vi "build_polymorphic_queues.vi"(2 "object/interaction_cluster_paths (in)":path[](array[path]), 5 "error in (no error)":errorcluster, 7 "base_federate_dir (in)":path, 8 "status_ref (in)":refnum<vi>) -> (19 "error out":errorcluster)   [LabVIEW 2016]
uses:
  controls/build_polymorphic_queues_actions.ctl
  <vilib>/picture/picture.llb/imagedata.ctl
  <vilib>/Utility/miscctls.llb/LVPositionTypeDef.ctl
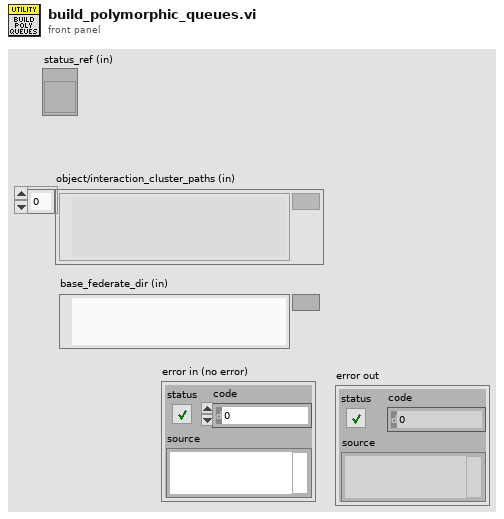
[diagram p1: front panel]
types:
  T1 = typedef "build_polymorphic_queues_actions.ctl" = enum16{"--------- unused ---------", "create_poly_instances", "create_poly_queues", "init"}
  T2 = typedef "imagedata.ctl" = cluster{"image type":i32, "image depth":i32, "image":u8[], "mask":u8[], "colors":u32[], "Rectangle":cluster{"left":i16, "top":i16, "right":i16, "bottom":i16}}
  T3 = enum32{"invalid app kind", "Development System", "Run Time System", "Student Edition", "Embedded LabVIEW", "Evaluation", "Custom"}
  T4 = typedef "LVPositionTypeDef.ctl" = cluster{"Left":i32, "Top":i32}
  T5 = enum32{"invalid VI type", "Standard VI", "Control VI", "Global VI", "Polymorphic VI", "Configuration VI", "SubSystem", "Facade VI", "Method VI", "Statechart Diagram VI"}
  T6 = cluster{"VIPath":path, "Menu Name":string, "Selector Name":string}
  T7 = cluster{"VIPath":path, "Menu Name":string, "Selector Name":string}[][]
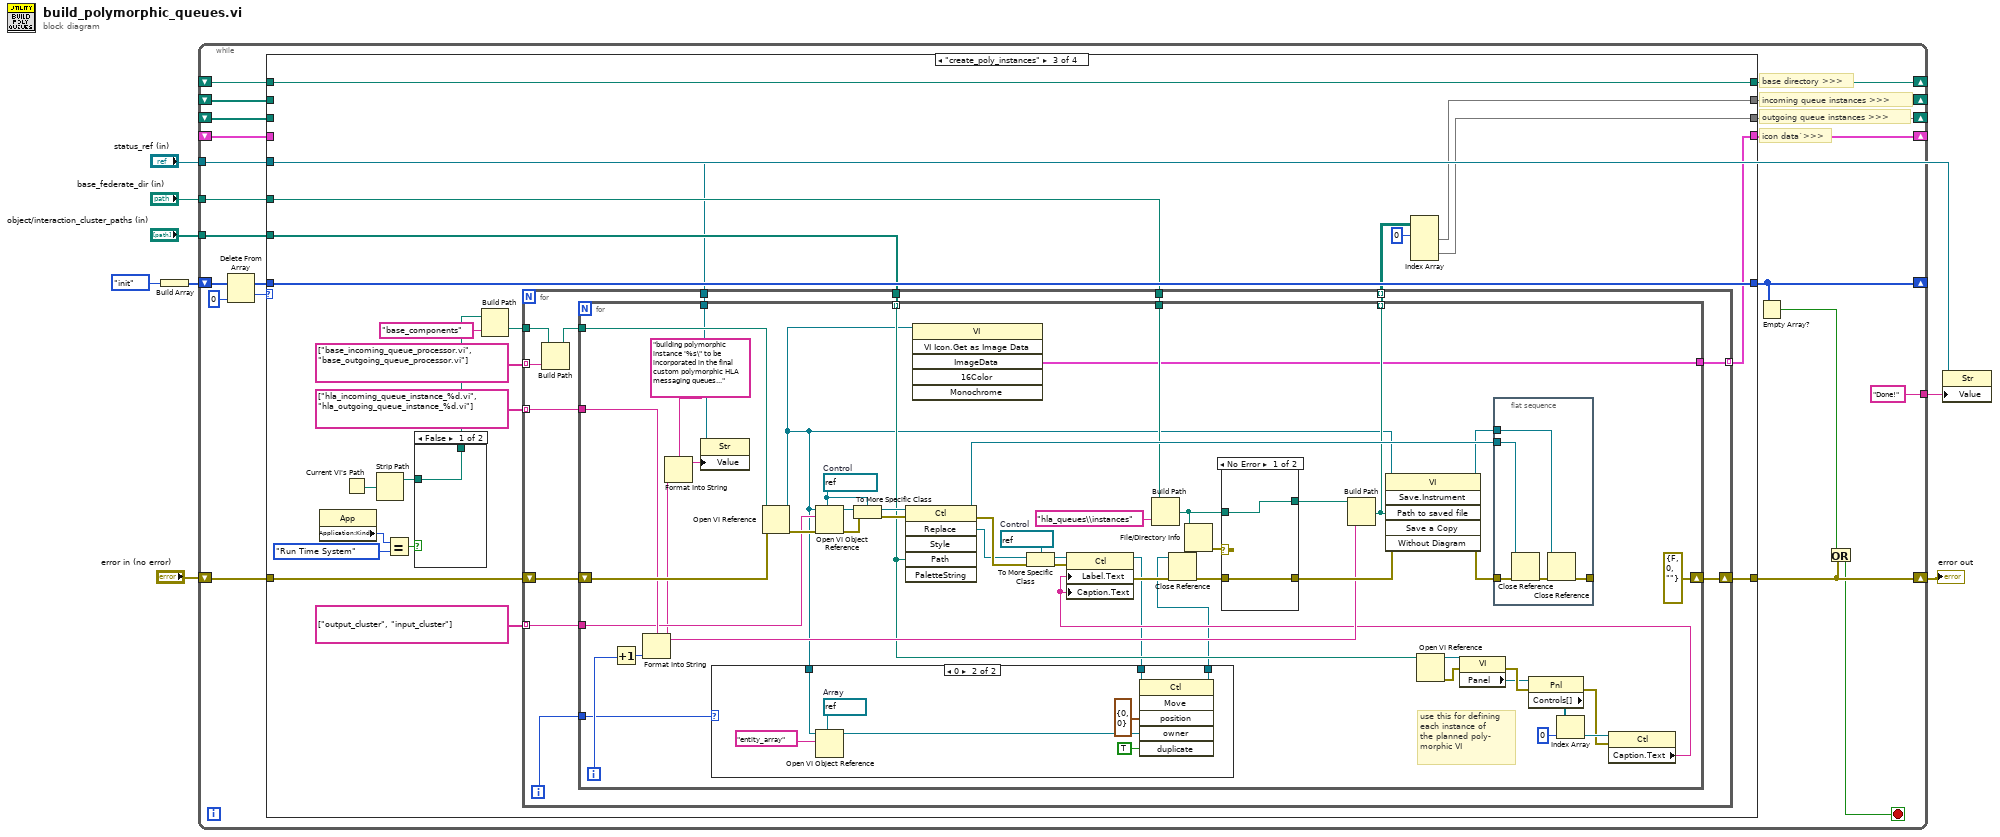
[diagram p0: block diagram]
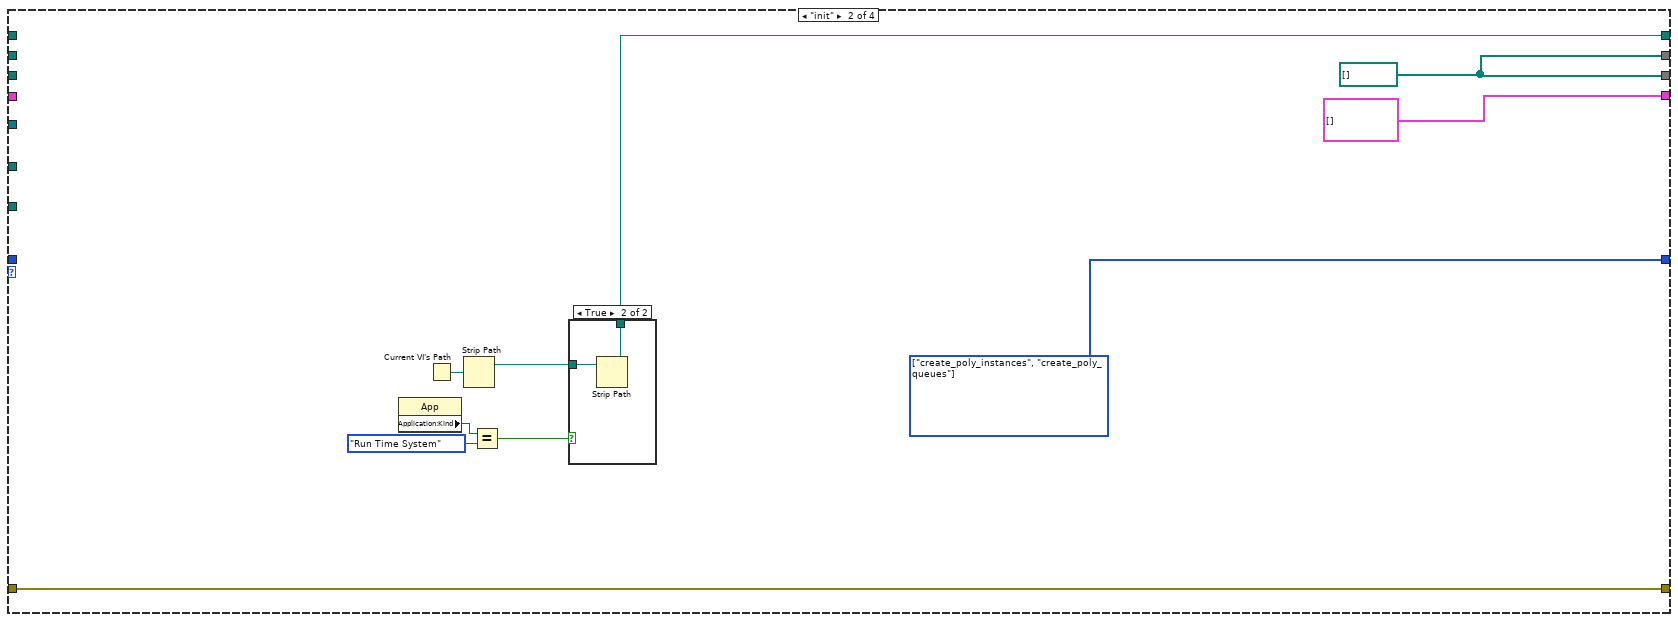
[diagram p3: hidden frame]
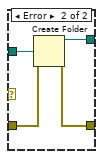
[diagram p6: hidden frame]
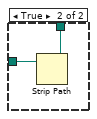
[diagram p7: hidden frame]
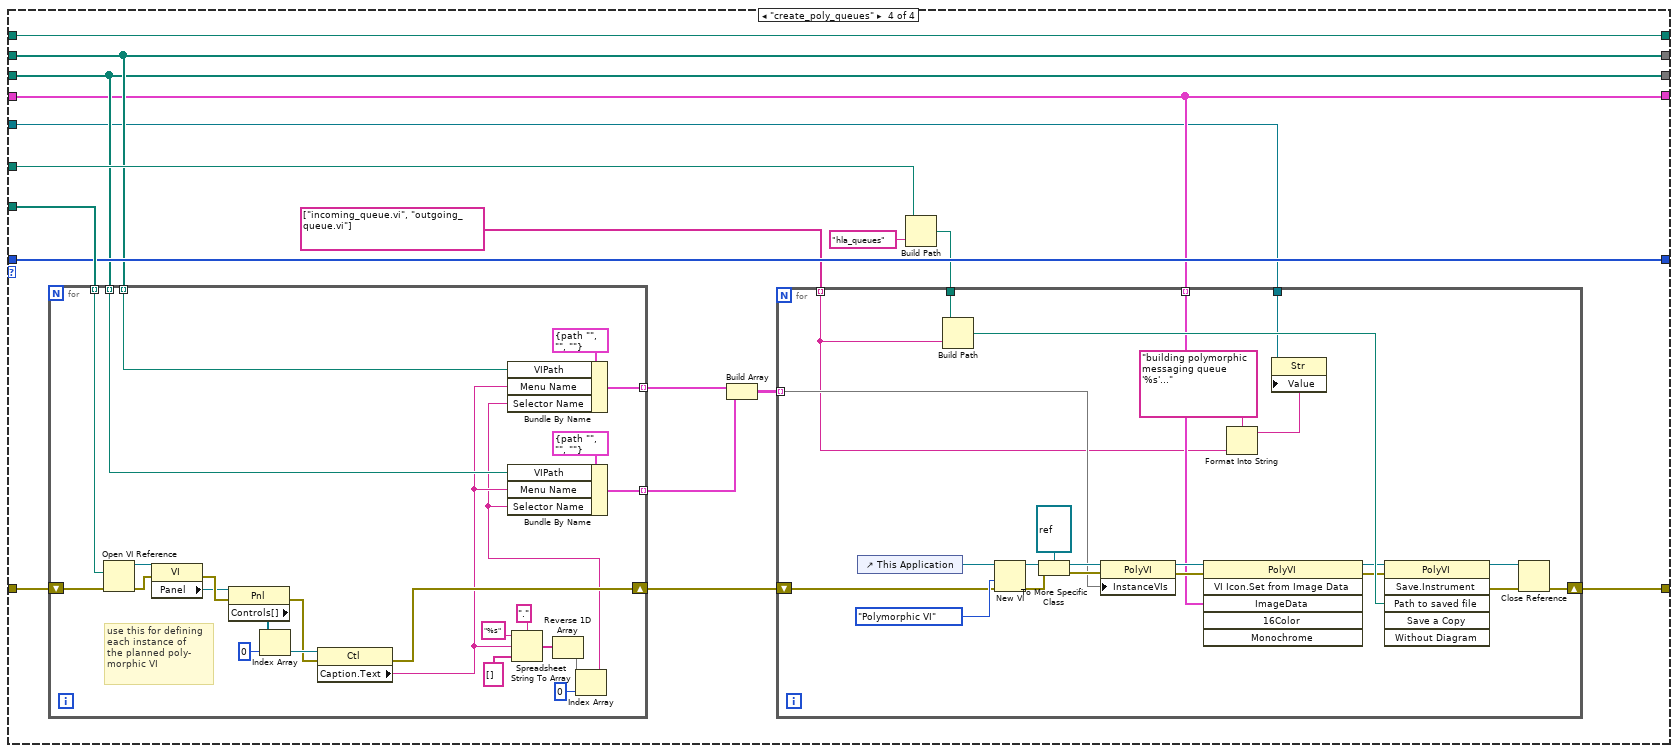
[diagram p8: hidden frame]
diagram:
  n1 = Build Array(build_polymorphic_queues_actions."init" ("actions")) -> (w7:T1[])
  n2 = while {
    shift-right: [w20] -> _
    shift-left: w7 -> [w29]
    shift-right: [w18] -> w6
    shift-left: "error in (no error)" -> [w26]
    shift-right: [w25] -> _
    shift-left: _ -> [w21]
    shift-right: [w23] -> _
    shift-left: _ -> [w22]
    shift-right: [w16] -> _
    shift-left: _ -> [w15]
    tunnel: "object/interaction_cluster_paths (in)" -> [w14]
    tunnel: "base_federate_dir (in)" -> [w13]
    shift-right: [w12] -> _
    shift-left: _ -> [w11]
    tunnel: "status_ref (in)" -> [w10]
    tunnel: ["Done!"] -> w1
    stop <- w17 stop-if-true
    # "icon data`>>>"
    # "outgoing queue instances >>>"
    # "incoming queue instances >>>"
    # "base directory >>>"
    n3 = Delete From Array(array=w29, index=0) -> (deleted portion=w27:T1, array with subset deleted=w24:T1[])  [unwired: 1 in]
    n4 = case shown="\"create_poly_instances\"" w27 {
      tunnel: [w32 w45 w71 w171] -> w20
      tunnel: w26 -> [w31 w44 w62 w172]
      tunnel: [w31 w44 w61 w162] -> w18
      tunnel: [w33 w37 w52 w160] -> w25
      tunnel: w24 -> [w32 _ w71 w171]
      tunnel: [w35 w38 w70 w170] -> w23
      tunnel: w22 -> [w35 _ w70 w170]
      tunnel: w21 -> [w33 _ _ w160]
      tunnel: [w34 w37 w53 w161] -> w16
      tunnel: w15 -> [w34 _ _ w161]
      tunnel: w14 -> [_ _ w58 w173]
      tunnel: w13 -> [_ _ w56 w165]
      tunnel: [w30 T2[] [] w50 w158] -> w12
      tunnel: w11 -> [w30 _ _ w158]
      tunnel: w10 -> [_ _ w49 w157]
      frame "--------- unused ---------" {
      }
      frame "init" {
        w37 = path[] []
        w45 = T1[] [enum."create_poly_instances", enum."create_poly_queues"] items=["--------- unused ---------", "create_poly_instances", "create_poly_queues", "init"]
        n5 = property on="Property Node" class="App"() -> ("Application:Kind"=w42:T3)  [unwired: 2 in, 2 out]
        n6 = Current VI's Path() -> (path=w43:path)
        n7 = Strip Path(path=w43) -> (stripped path=w39:path)  [unwired: 1 out]
        n8 = Equal?(x=w42, y=T3."Run Time System") -> (x = y?=w40:bool)
        n9 = case shown="True" w40 {
          tunnel: w39 -> [w46 w48]
          tunnel: [w46 w47] -> w38
          frame False {
          }
          frame True {
            n10 = Strip Path(path=w48) -> (stripped path=w47:path)  [unwired: 1 out]
          }
        }
      }
      frame "create_poly_instances" {
        n11 = property on="Property Node" class="App"() -> ("Application:Kind"=w66:T3)  [unwired: 2 in, 2 out]
        n12 = Current VI's Path() -> (path=w65:path)
        n13 = Strip Path(path=w65) -> (stripped path=w69:path)  [unwired: 1 out]
        n14 = Equal?(x=w66, y=T3."Run Time System") -> (x = y?=w68:bool)
        n15 = case shown="False" w68 {
          tunnel: w69 -> [w154 w156]
          tunnel: [w154 w155] -> w64
          frame False {
          }
          frame True {
            n16 = Strip Path(path=w156) -> (stripped path=w155:path)  [unwired: 1 out]
          }
        }
        n17 = Build Path(base path=w64, name or relative path="base_components") -> (appended path=w60:path)
        n18 = for {
          shift-right: [w81] -> w61
          shift-left: w62 -> [w82]
          tunnel: w60 -> [w84]
          tunnel: string[] ["base_incoming_queue_processor.vi", "base_outgoing_queue_processor.vi"] -> [w83] mode=indexing
          tunnel: w58 -> [w80]
          tunnel: string[] ["hla_incoming_queue_instance_%d.vi", "hla_outgoing_queue_instance_%d.vi"] -> [w74] mode=indexing
          tunnel: w56 -> [w78]
          tunnel: [w77] -> w55 mode=indexing
          tunnel: string[] ["output_cluster", "input_cluster"] -> [w76] mode=indexing
          tunnel: [w75] -> w50 mode=indexing
          tunnel: w49 -> [w73]
          i -> [w72]
          n19 = Build Path(base path=w84, name or relative path=w83) -> (appended path=w79:path)
          n20 = for {
            shift-right: [errorcluster {"status"=FALSE, "code"=0, "source"=""} ("error in (no error)")] -> w81
            shift-left: w82 -> [w113]
            tunnel: w80 -> [w91] mode=indexing
            tunnel: w74 -> [w110]
            tunnel: w79 -> [w109]
            tunnel: w78 -> [w108]
            tunnel: [w107] -> w77 mode=indexing
            tunnel: w76 -> [w106]
            tunnel: [w104] -> w75
            tunnel: w73 -> [w101]
            tunnel: w72 -> [w85]
            i -> [w112]
            w119 = refnum<vi> refnum  # Control
            w115 = refnum<vi> refnum  # Control
            # "use this for defining\neach instance of\nthe planned poly-\nmorphic VI"
            n21 = Increment(x=w112) -> (x+1=w111:i32)
            n22 = Format Into String(format string=w110, w111) -> (resulting string=w100:string)  [unwired: 2 in, 1 out]
            n23 = Format Into String(format string="building polymorphic instance '%s\" to be incorporated in the final custom polymorphic HLA messaging queues...", w100) -> (resulting string=w103:string)  [unwired: 2 in, 1 out]
            n24 = property class="Str"(reference=w101, "Value"=w103) -> ()  [unwired: 1 in, 2 out]
            n25 = Open VI Reference(vi path=w109, error in (no error)=w113) -> (vi reference=w89:refnum<vi>, error out=w126:errorcluster)  [unwired: 4 in]
            n26 = Open VI Object Reference(7:w115, 8:w126, 10:w106, 11:w89) -> (0:w121:errorcluster, 3:w114:refnum<vi>)
            n27 = To More Specific Class(target class=w115, reference=w114, error in=w121) -> (specific class reference=w116:refnum<vi>, error out=w122:errorcluster)
            n28 = invoke class="Ctl" method="Replace"(reference=w116, error in=w122, "Path"=w91) -> (reference out=w118:refnum<vi>, error out=w124:errorcluster, "Replace"=w88:refnum<vi>)  [unwired: 3 in, 3 out]
            n29 = invoke class="VI" method="VI Icon.Get as Image Data"(reference=w89) -> ("ImageData"=w104:T2)  [unwired: 5 in, 5 out]
            n30 = To More Specific Class(target class=w119, reference=w88, error in=w124) -> (specific class reference=w120:refnum<vi>, error out=w123:errorcluster)
            n31 = Build Path(base path=w108, name or relative path="hla_queues\\instances") -> (appended path=w128:path)
            n32 = File/Directory Info(path=w128) -> (error out=w127:errorcluster)  [unwired: 1 in, 6 out]
            n33 = Open VI Reference(vi path=w91) -> (vi reference=w93:refnum<vi>, error out=w92:errorcluster)  [unwired: 5 in]
            n34 = property class="VI"(reference=w93, error in=w92) -> (error out=w97:errorcluster, "Panel"=w94:refnum<vi>)  [unwired: 1 out]
            n35 = flat-sequence {
              tunnel: w117 -> [w153]
              tunnel: w118 -> [w152]
              tunnel: w133 -> [w151]
              tunnel: [w149] -> _
              frame #0 {
                n36 = Close Reference(reference=w152, error in (no error)=w151) -> (error out=w150:errorcluster)
                n37 = Close Reference(reference=w153, error in (no error)=w150) -> (error out=w149:errorcluster)
              }
            }
            n38 = property class="Pnl"(reference=w94, error in=w97) -> (error out=w98:errorcluster, "Controls[]"=w95:refnum<vi>[])  [unwired: 1 out]
            n39 = Index Array(array=w95, index=0) -> (element=w99:refnum<vi>)
            n40 = property class="Ctl"(reference=w99, error in=w98) -> ("Caption.Text"=w90:string)  [unwired: 2 out]
            n41 = property class="Ctl"(reference=w120, error in=w123, "Label.Text"=w90, "Caption.Text"=w90) -> (reference out=w87:refnum<vi>, error out=w125:errorcluster)
            n42 = case shown="0" w85 {
              tunnel: w89 -> [_ w141]
              tunnel: w87 -> [w134 w137]
              tunnel: [w134 w136] -> w86
              frame Default {
              }
              frame 0 {
                w142 = refnum<vi> refnum  # Array
                n43 = Open VI Object Reference(7:w142, 10:"entity_array", 11:w141) -> (3:w138:refnum<vi>)  [unwired: 1 in, 1 out]
                n44 = invoke class="Ctl" method="Move"(reference=w137, "position"=T4 {"Left"=0, "Top"=0}, "owner"=w138, "duplicate"=TRUE ("Duplicate? (F)")) -> (reference out=w136:refnum<vi>)  [unwired: 2 in, 5 out]
              }
            }
            n45 = Close Reference(reference=w86, error in (no error)=w125) -> (error out=w130:errorcluster)
            n46 = case shown="No Error" w127 {
              tunnel: w130 -> [w143 w148]
              tunnel: [w143 w147] -> w132
              tunnel: [w144 w146] -> w131
              tunnel: w128 -> [w144 w145]
              frame No Error {
              }
              frame Error {
                n47 = Create Folder(path (use dialog)=w145, error in=w148) -> (created path=w146:path, error out=w147:errorcluster)  [unwired: 1 in, 1 out]
              }
            }
            n48 = Build Path(base path=w131, name or relative path=w100) -> (appended path=w107:path)
            n49 = invoke class="VI" method="Save.Instrument"(reference=w89, error in=w132, "Path to saved file"=w107) -> (reference out=w117:refnum<vi>, error out=w133:errorcluster)  [unwired: 3 in, 4 out]
          }
        }
        n50 = Index Array(array=w55, index (row) #1=0 ("index (row)")) -> (element #1=w53:path[], element #2=w52:path[])  [unwired: 3 in]
      }
      frame "create_poly_queues" {
        n51 = for {
          tunnel: w160 -> [w216] mode=indexing
          tunnel: w161 -> [w217] mode=indexing
          tunnel: w173 -> [w221] mode=indexing
          shift-right: [w205] -> w167
          shift-left: w172 -> [w220]
          tunnel: [w215] -> w169 mode=indexing
          tunnel: [w214] -> w168 mode=indexing
          # "use this for defining\neach instance of\nthe planned poly-\nmorphic VI"
          n52 = Open VI Reference(vi path=w221, error in (no error)=w220) -> (vi reference=w207:refnum<vi>, error out=w206:errorcluster)  [unwired: 4 in]
          n53 = property class="VI"(reference=w207, error in=w206) -> (error out=w211:errorcluster, "Panel"=w208:refnum<vi>)  [unwired: 1 out]
          n54 = property class="Pnl"(reference=w208, error in=w211) -> (error out=w212:errorcluster, "Controls[]"=w209:refnum<vi>[])  [unwired: 1 out]
          n55 = Index Array(array=w209, index=0) -> (element=w213:refnum<vi>)
          n56 = property class="Ctl"(reference=w213, error in=w212) -> (error out=w205:errorcluster, "Caption.Text"=w202:string)  [unwired: 1 out]
          n57 = Spreadsheet String To Array(delimiter (Tab)=".", format string="%s", spreadsheet string=w202, array type (2D Dbl)=string[] []) -> (array=w200:string[])
          n58 = Reverse 1D Array(array=w200) -> (reversed array=w199:string[])
          n59 = Index Array(array=w199, index=0) -> (element=w197:string)
          n60 = Bundle By Name(cluster=T6 {"VIPath"=path "", "Menu Name"="", "Selector Name"=""}, "VIPath"=w217, "Menu Name"=w202, "Selector Name"=w197) -> (w215:T6)
          n61 = Bundle By Name(cluster=T6 {"VIPath"=path "", "Menu Name"="", "Selector Name"=""}, "VIPath"=w216, "Menu Name"=w202, "Selector Name"=w197) -> (w214:T6)
        }
        n62 = Build Array(w169, w168) -> (w159:T7)
        n63 = Build Path(base path=w165, name or relative path="hla_queues") -> (appended path=w164:path)
        n64 = for {
          shift-right: [w186] -> w162
          shift-left: w167 -> [w187]
          tunnel: w164 -> [w185]
          tunnel: string[] ["incoming_queue.vi", "outgoing_queue.vi"] -> [w175] mode=indexing
          tunnel: w159 -> [w183] mode=indexing
          tunnel: w158 -> [w178] mode=indexing
          tunnel: w157 -> [w177]
          n65 = control-ref of="This Application"() -> (w188:refnum<vi>)
          n66 = Build Path(base path=w185, name or relative path=w175) -> (appended path=w184:path)
          n67 = New VI(8:w187, 9:T5."Polymorphic VI" ("vi type (standard vi)"), 11:w188) -> (0:w195:errorcluster, 3:w191:refnum<vi>)  [unwired: 4 in]
          n68 = To More Specific Class(target class=refnum<vi> refnum ("vi refnum"), reference=w191, error in=w195) -> (specific class reference=w192:refnum<vi>, error out=w196:errorcluster)
          n69 = property class="PolyVI"(reference=w192, error in=w196, "InstanceVIs"=w183) -> (reference out=w180:refnum<vi>, error out=w182:errorcluster)
          n70 = invoke class="PolyVI" method="VI Icon.Set from Image Data"(reference=w180, error in=w182, "ImageData"=w178) -> (reference out=w179:refnum<vi>, error out=w181:errorcluster)  [unwired: 3 in, 4 out]
          n71 = Format Into String(format string="building polymorphic messaging queue '%s'...", w175) -> (resulting string=w174:string)  [unwired: 2 in, 1 out]
          n72 = property class="Str"(reference=w177, "Value"=w174) -> ()  [unwired: 1 in, 2 out]
          n73 = invoke class="PolyVI" method="Save.Instrument"(reference=w179, error in=w181, "Path to saved file"=w184) -> (reference out=w193:refnum<vi>, error out=w194:errorcluster)  [unwired: 3 in, 4 out]
          n74 = Close Reference(reference=w193, error in (no error)=w194) -> (error out=w186:errorcluster)
        }
      }
    }
    n75 = Empty Array?(array=w20) -> (empty?=w19:bool)
    n76 = Or(x=w19, y=w18) -> (x .or. y?=w17:bool)
  }
  "error out" <- w6
  n77 = property class="Str"(reference="status_ref (in)", "Value"=w1) -> ()  [unwired: 1 in, 2 out]
